vi "q3 whitespace count.vi"() -> ()   [LabVIEW 2025]
panel:
  out "Count":dbl
  in  "String":string
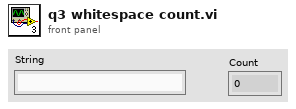
[diagram p1: front panel]
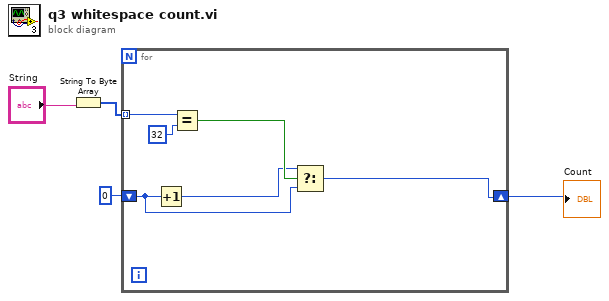
[diagram p0: block diagram]
diagram:
  n1 = String To Byte Array(string="String") -> (unsigned byte array=w3:u8[])
  n2 = for {
    tunnel: w3 -> [w10] mode=indexing
    shift-right: [w5] -> w1
    shift-left: 0 -> [w6]
    n3 = Increment(x=w6) -> (x+1=w7:i32)
    n4 = Equal?(x=w10, y=32) -> (x = y?=w8:bool)
    n5 = Select(t=w7, s=w8, f=w6) -> (s? t:f=w5:i32)
  }
  "Count" <- w1
